vi "Open Settings Dialog.vi"(8 "error in (no error)":errorcluster, 11 "HIJ Vision Camera App in":refnum<class "HIJ Vision Camera App.lvclass">) -> (0 "error out":errorcluster, 3 "HIJ Vision Camera App out":refnum<class "HIJ Vision Camera App.lvclass">)   [LabVIEW 2014, in "HIJ Vision Camera App.lvlib" / "HIJ Vision Camera App.lvclass"]
uses:
  HIJ Vision Camera App.lvclass
  HIJ Vision Camera App.lvclass/HIJ Vision Camera App.ctl
  <vilib>/ActorFramework/Message Enqueuer/Message Enqueuer.lvclass/Message Enqueuer.ctl
  <vilib>/ActorFramework/Message Enqueuer/Enqueue.vi
  <vilib>/ActorFramework/Message Priority Queue/Priority Enqueue.vi
  Shared Code/Viewable Actor/ViewableActor Messages/Open Front Panel Msg/Open Front Panel Msg.lvclass
  <vilib>/ActorFramework/Actor/Actor.lvclass
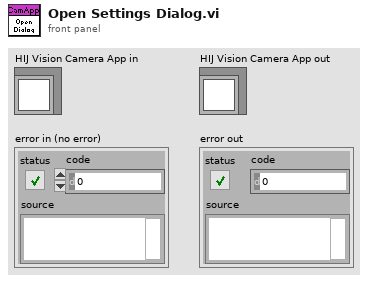
[diagram p1: front panel]
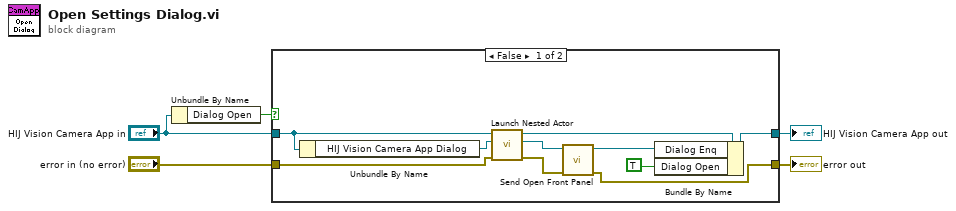
[diagram p0: block diagram]
diagram:
  n1 = Unbundle By Name("HIJ Vision Camera App in") -> ("Dialog Open"=w1:bool)
  n2 = case shown="False" w1 {
    tunnel: [w9 w17] -> w2
    tunnel: "HIJ Vision Camera App in" -> [w15 w17]
    tunnel: "error in (no error)" -> [w12 w16]
    tunnel: [w10 w16] -> w5
    frame False {
      n3 = Unbundle By Name(w15) -> ("HIJ Vision Camera App Dialog"=w13:refnum<class "HIJ Vision Camera App Dialog.lvclass">)
      n4 = call <vilib>:"Launch Nested Actor.vi"("error in (no error)"=w12, "Nested Actor"=w13, "Caller Actor in"=w15) -> ("error out"=w11:errorcluster, "Nested Actor's Enqueuer"=w8:refnum<class "Message Enqueuer.lvclass">, "Caller Actor out"=w14:refnum<class "HIJ Vision Camera App.lvclass">)  [unwired: 6 in]
      n5 = call "Send Open Front Panel.vi"("error in (no error)"=w11, "Message Enqueuer"=w8) -> ("error out"=w10:errorcluster, "Message Enqueuer out"=w7:refnum<class "Message Enqueuer.lvclass">)  [unwired: 8 in]
      n6 = Bundle By Name(cluster=w14, "Dialog Enq"=w7, "Dialog Open"=TRUE) -> (w9:refnum<class "HIJ Vision Camera App.lvclass">)
    }
    frame True {
    }
  }
  "error out" <- w5
  "HIJ Vision Camera App out" <- w2
